vi "Check if Gold Board.vi"(8 "error in (no error)":errorcluster, 10 "Serial Number":string, 11 "Golden Board in":refnum<class "Golden Board.lvclass">) -> (0 "error out":errorcluster, 1 "GoldSerNos":string[](array[string]), 2 "Gold Board":bool, 3 "Golden Board out":refnum<class "Golden Board.lvclass">, 5 "Material Name":string)   [LabVIEW 2017, in "Golden Board.lvlib" / "Golden Board.lvclass"]
doc: "Compares the incoming LotID against the Gold Board file to see if it is (or part of) a gold board. If \"Gold Board\" returns a TRUE value, \"Material Name\" and \"GoldSerNos\" will be populated with the appropriate values. If LotID is part of a panel of gold boards than GoldSerNos will return an array of values in position order of Golden Serial Numbers."
uses:
  Golden Board.lvclass
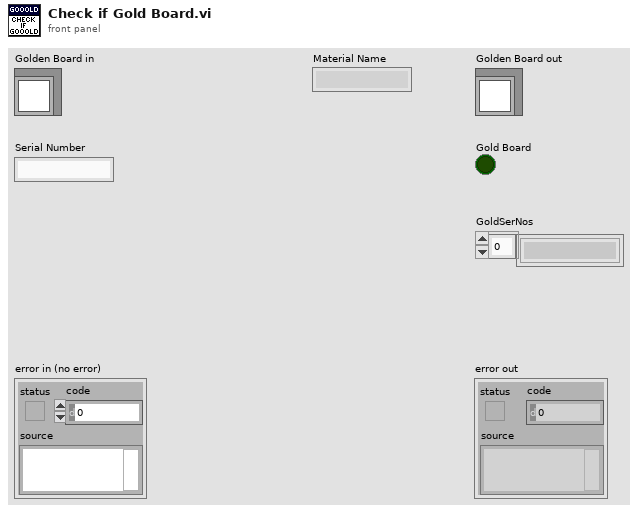
[diagram p1: front panel]
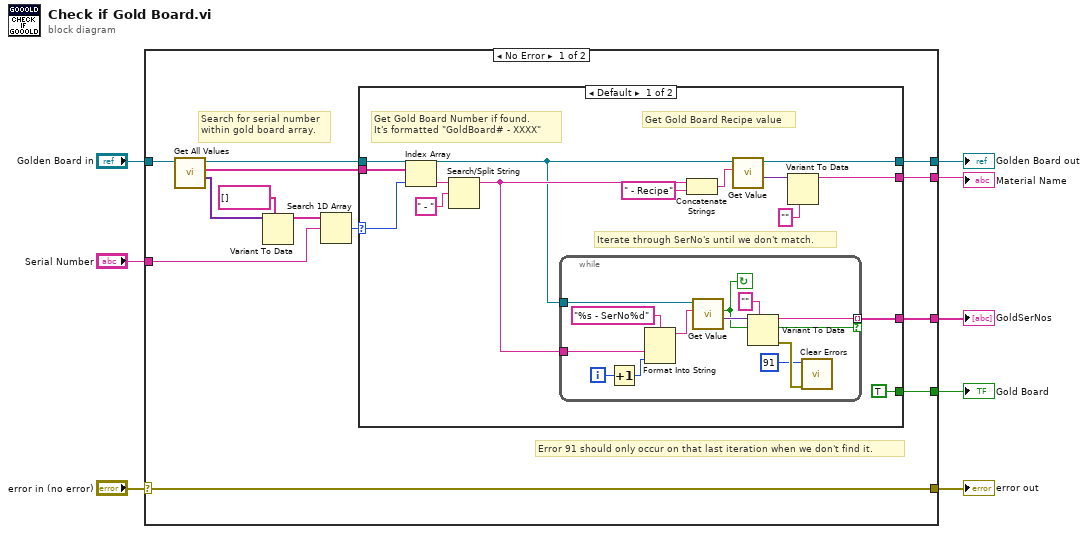
[diagram p0: block diagram]
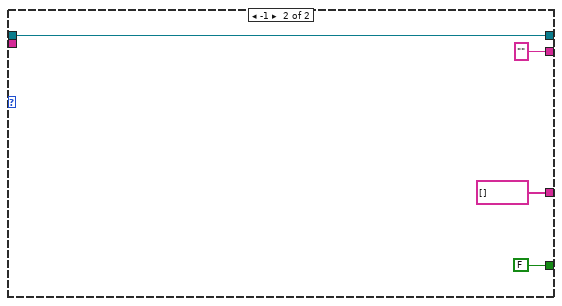
[diagram p2: hidden frame]
diagram:
  n1 = case shown="No Error" "error in (no error)" {
    selector: "error in (no error)" -> [w10 w53]
    tunnel: "Serial Number" -> [w21 _]
    tunnel: [w20 _] -> w1
    tunnel: [w19 _] -> w2
    tunnel: [w18 _] -> w3
    tunnel: "Golden Board in" -> [w11 w52]
    tunnel: [w10 w53] -> w7
    tunnel: [w9 w52] -> w5
    frame No Error {
      # "Error 91 should only occur on that last iteration when we don't find it."
      # "Search for serial number\nwithin gold board array."
      n2 = call-dynamic "Get All Values.vi"("Registry in"=w11) -> ("Values"=w16:variant[], "Keys"=w13:string[], "Registry out"=w12:refnum<class "Golden Board.lvclass">)  [unwired: 7 in, 1 out]
      n3 = Variant To Data(type=string[] [], Variant=w16) -> (data=w15:string[])  [unwired: 1 in, 1 out]
      n4 = Search 1D Array(1D array=w15, element=w21) -> (index of element=w14:i32)  [unwired: 1 in]
      n5 = case shown="Default" w14 {
        selector: w14 -> [w33 _]
        tunnel: [TRUE FALSE] -> w20
        tunnel: [w26 "" ("Key Value")] -> w18
        tunnel: [w24 string[] [] ("GoldSerNos")] -> w19
        tunnel: w13 -> [w34 _]
        tunnel: w12 -> [w23 w48]
        tunnel: [w22 w48] -> w9
        frame Default {
          # "Iterate through SerNo's until we don't match."
          # "Get Gold Board Recipe value"
          # "Get Gold Board Number if found.\nIt's formatted \"GoldBoard# - XXXX\""
          n6 = Index Array(array=w34, index=w33) -> (element=w32:string)
          n7 = Search/Split String(string=w32, search string/char (-)=" - ") -> (substring before match=w25:string)  [unwired: 1 in, 2 out]
          n8 = while {
            tunnel: [w45] -> w24 mode=indexing if=w38
            tunnel: w25 -> [w40]
            tunnel: w23 -> [w37]
            i -> [w44]
            stop <- w38 continue-if-true
            n9 = Increment(x=w44) -> (x+1=w41:i32)
            n10 = Format Into String(format string="%s - SerNo%d", w40, w41) -> (resulting string=w43:string)  [unwired: 2 in, 1 out]
            n11 = call-dynamic "Get Value.vi"("Key"=w43, "Registry in"=w37) -> ("Value"=w46:variant, "found?"=w38:bool)  [unwired: 6 in, 2 out]
            n12 = Variant To Data(type="" ("search string/char (-)"), Variant=w46) -> (data=w45:string, error out=w39:errorcluster)  [unwired: 1 in]
            n13 = call <vilib>:"Clear Errors.vi"("error in (no error)"=w39, "specific error code to clear (0: all)"=91) -> ()  [unwired: 4 in, 2 out]
          }
          n14 = Concatenate Strings(w25, " - Recipe" ("search string/char (-)")) -> (w29:string)
          n15 = call-dynamic "Get Value.vi"("Key"=w29, "Registry in"=w23) -> ("Value"=w28:variant, "Registry out"=w22:refnum<class "Golden Board.lvclass">)  [unwired: 6 in, 2 out]
          n16 = Variant To Data(type="" ("search string/char (-)"), Variant=w28) -> (data=w26:string)  [unwired: 1 in, 1 out]
        }
        frame -1 {
        }
      }
    }
    frame Error {
    }
  }
  "error out" <- w7
  "Golden Board out" <- w5
  "Material Name" <- w3
  "GoldSerNos" <- w2
  "Gold Board" <- w1
